vi "起始时间.vi"() -> ()   [LabVIEW 2016]
panel:
  out "结束时间":string
  out "起始时间":string
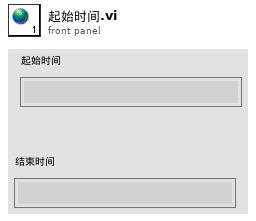
[diagram p1: front panel]
diagram:
